vi "Rings.vi"(8 "error in (no error)":errorcluster, 11 "Rings":i32) -> (0 "error out":errorcluster)   [LabVIEW 2015]
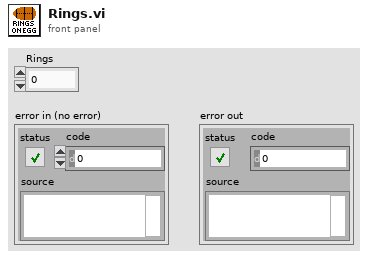
[diagram p1: front panel]
types:
  T1 = cluster{"MS1 (A/DIO1 (Pin 13))":bool, "MS2 (A/DIO2 (Pin 15))":bool, "MS3 (A/DIO3 (Pin 17))":bool}
  T2 = cluster{"MS1 (C/DIO5 (DIO5))":bool, "MS2 (C/DIO6 (DIO6))":bool, "MS3 (C/DIO7 (DIO7))":bool}
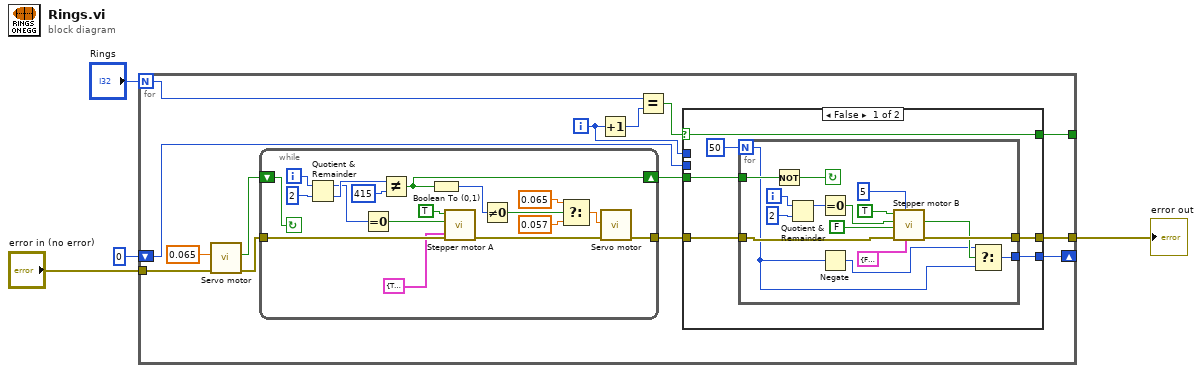
[diagram p0: block diagram]
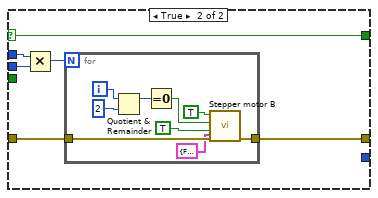
[diagram p2: hidden frame]
diagram:
  n1 = for {
    N: "Rings" -> [w10]
    tunnel: [w18] -> w1
    shift-right: [w9] -> _
    shift-left: 0 -> [w8]
    tunnel: "error in (no error)" -> [w6]
    tunnel: [w5] -> _
    i -> [w7]
    n2 = call "Servo motor.vi"("error in (no error)"=w6, "Duty Cycle"=0.065) -> ("error out"=w16:errorcluster, "Drop?"=w17:bool)  [unwired: 8 in]
    n3 = while {
      shift-right: [w66] -> w13
      shift-left: w17 -> [w67]
      tunnel: [w58] -> w15
      tunnel: w16 -> [w65]
      i -> [w72]
      stop <- w67 continue-if-true
      n4 = Quotient & Remainder(x=w72, y=2) -> (x-y*floor(x/y)=w56:i32, floor(x/y)=w69:i32)
      n5 = Equal To 0?(x=w56) -> (x = 0?=w70:bool)
      n6 = Not Equal?(x=w69, y=415) -> (x != y?=w66:bool)
      n7 = Boolean To (0,1)(Boolean=w66) -> (0, 1=w64:i16)
      n8 = call "Stepper motor A.vi"("Microstep size"=T2 {"MS1 (C/DIO5 (DIO5))"=TRUE, "MS2 (C/DIO6 (DIO6))"=FALSE, "MS3 (C/DIO7 (DIO7))"=FALSE} ("Microstepping"), "error in (no error)"=w65, "Step (C/DIO3 (DIO3))"=w70, "Enable (C/DIO2 (DIO2))"=TRUE) -> ("error out"=w59:errorcluster)  [unwired: 7 in]
      n9 = Not Equal To 0?(x=w64) -> (x != 0?=w63:bool)
      n10 = Select(t=0.065, s=w63, f=0.057) -> (s? t:f=w62:dbl)
      n11 = call "Servo motor.vi"("error in (no error)"=w59, "Duty Cycle"=w62) -> ("error out"=w58:errorcluster)  [unwired: 8 in, 1 out]
    }
    n12 = Increment(x=w7) -> (x+1=w12:i32)
    n13 = Equal?(x=w10, y=w12) -> (x = y?=w11:bool)
    n14 = case shown="False" w11 {
      selector: w11 -> [w19 w41]
      tunnel: [w24 w45] -> w18
      tunnel: w15 -> [w22 w46]
      tunnel: w13 -> [w21 _]
      tunnel: w7 -> [_ w44]
      tunnel: [w20 _] -> w9
      tunnel: w8 -> [_ w42]
      tunnel: [w19 w41] -> w5
      frame False {
        n15 = for {
          N: 50 ("Numeric Control") -> [w26]
          tunnel: w22 -> [w34]
          tunnel: [w33] -> w24
          tunnel: w21 -> [w30]
          tunnel: [w25] -> w20
          i -> [w36]
          stop <- w35 continue-if-true
          n16 = Not(x=w30) -> (.not. x?=w35:bool)
          n17 = Quotient & Remainder(x=w36, y=2) -> (x-y*floor(x/y)=w38:i32)  [unwired: 1 out]
          n18 = Equal To 0?(x=w38) -> (x = 0?=w37:bool)
          n19 = Negate(x=w26) -> (-x=w27:i32)
          n20 = call "Stepper motor B.vi"("Microstep size"=T1 {"MS1 (A/DIO1 (Pin 13))"=FALSE, "MS2 (A/DIO2 (Pin 15))"=TRUE, "MS3 (A/DIO3 (Pin 17))"=FALSE} ("Microstepping"), "Speed"=u32 5, "error in (no error)"=w34, "Direction (A/DIO5 (Pin 21))"=FALSE, "Step (A/DIO4 (Pin 19))"=w37, "Enable (A/DIO0 (Pin 11))"=TRUE) -> ("error out"=w33:errorcluster, "Direction"=w28:bool)  [unwired: 4 in]
          n21 = Select(t=w27, s=w28, f=w26) -> (s? t:f=w25:i32)
        }
      }
      frame True {
        n22 = Multiply(x=w44, y=w42) -> (x*y=w43:i32)
        n23 = for {
          N: w43 -> [_]
          tunnel: w46 -> [w54]
          tunnel: [w53] -> w45
          i -> [w52]
          n24 = Quotient & Remainder(x=w52, y=2) -> (x-y*floor(x/y)=w50:i32)  [unwired: 1 out]
          n25 = Equal To 0?(x=w50) -> (x = 0?=w49:bool)
          n26 = call "Stepper motor B.vi"("Microstep size"=T1 {"MS1 (A/DIO1 (Pin 13))"=FALSE, "MS2 (A/DIO2 (Pin 15))"=TRUE, "MS3 (A/DIO3 (Pin 17))"=FALSE} ("Microstepping"), "error in (no error)"=w54, "Direction (A/DIO5 (Pin 21))"=TRUE, "Step (A/DIO4 (Pin 19))"=w49, "Enable (A/DIO0 (Pin 11))"=TRUE) -> ("error out"=w53:errorcluster)  [unwired: 5 in, 1 out]
        }
      }
    }
  }
  "error out" <- w1
